vi "createLogFile (SubVI).vi"(8 "TrialInfo":T2={"BlockInfo"={"block #"=0, "block cond"=enum."RHP", "Trial # in block"=0}, "Trial #"=0}, 10 "Subject ID":T1, 11 "directory Path":path) -> (3 "file path out":path)   [LabVIEW 2021]
uses:
  ctrTrialInfo.ctl
  ctrBlockInfo.ctl
  ctrBlockCondition.ctl
  ctlProtocolSubID.ctl
  ctrUnpredictpair.ctl
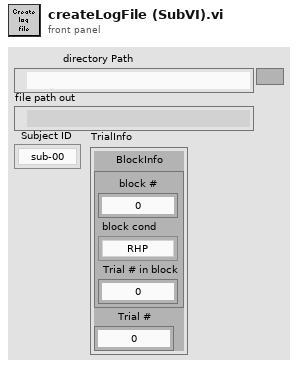
[diagram p1: front panel]
types:
  T1 = typedef "ctlProtocolSubID.ctl" = enum16{"sub-00", "sub-01", "sub-02", "sub-03", "sub-04", "sub-05", "sub-06", "sub-07", "sub-08", "sub-09", "sub-10", "sub-11", "sub-12", "sub-13", "sub-14", "sub-15", "sub-16", "sub-17", "sub-18", "sub-19", "sub-20", "sub-21", "sub-22", "sub-23", "sub-24", "sub-25", "sub-26", "sub-27", "sub-28", "sub-29", "sub-30", "sub-31", "sub-32", "sub-33", "sub-34", "sub-35", "sub-36", "sub-37", "sub-38", "sub-39", "sub-40"}
  T2 = typedef "ctrTrialInfo.ctl" = cluster{"BlockInfo":T3, "Trial #":i32}
  T3 = typedef "ctrBlockInfo.ctl" = cluster{"block #":i32, "block cond":T4, "Trial # in block":i32}
  T4 = typedef "ctrBlockCondition.ctl" = enum16{"famDrop", "preDrop", "famTask", "RHP", "RLD", "RHD", "LHP", "LLD", "LHD", "UR", "UL", "pstDrop"}
  T5 = typedef "ctrUnpredictpair.ctl" = enum16{"HPHP", "LDHP", "HDHP", "HPLD", "HPHD", "LDLD", "HDHD", "HP"}
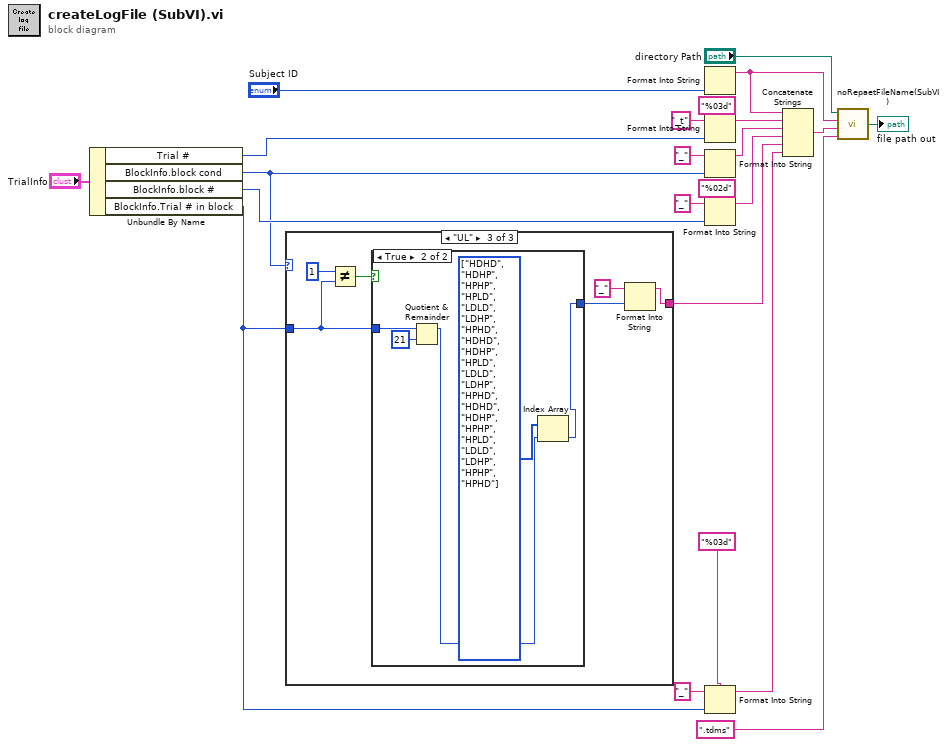
[diagram p0: block diagram]
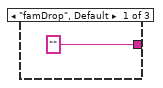
[diagram p2: hidden frame]
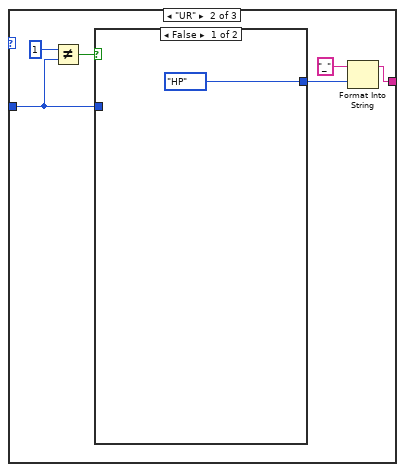
[diagram p3: hidden frame]
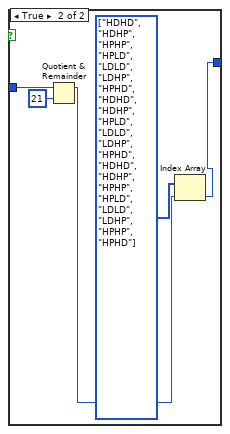
[diagram p4: hidden frame]
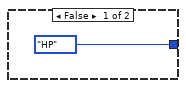
[diagram p5: hidden frame]
diagram:
  n1 = Unbundle By Name("TrialInfo") -> ("Trial #"=w4:i32, "BlockInfo.block cond"=w3:T4, "BlockInfo.block #"=w6:i32, "BlockInfo.Trial # in block"=w1:i32)
  n2 = case shown="\"UL\"" w3 {
    tunnel: ["" ("string") w25 w37] -> w2
    tunnel: w1 -> [_ w30 w42]
    frame "famDrop", Default {
    }
    frame "UR" {
      n3 = Not Equal?(x=1, y=w30) -> (x != y?=w28:bool)
      n4 = case shown="False" w28 {
        tunnel: w30 -> [_ w35]
        tunnel: [ctrUnpredictpair."HP" w32] -> w26
        frame False {
        }
        frame True {
          w34 = T5[] [enum."HDHD", enum."HDHP", enum."HPHP", enum."HPLD", enum."LDLD", enum."LDHP", enum."HPHD", enum."HDHD", enum."HDHP", enum."HPLD", enum."LDLD", enum."LDHP", enum."HPHD", enum."HDHD", enum."HDHP", enum."HPHP", enum."HPLD", enum."LDLD", enum."LDHP", enum."HPHP", enum."HPHD"] items=["HPHP", "LDHP", "HDHP", "HPLD", "HPHD", "LDLD", "HDHD", "HP"] ("Array")
          n5 = Quotient & Remainder(x=w35, y=21) -> (x-y*floor(x/y)=w33:i32)  [unwired: 1 out]
          n6 = Index Array(array=w34, index=w33) -> (element=w32:T5)
        }
      }
      n7 = Format Into String(initial string="_" ("string"), w26) -> (resulting string=w25:string)  [unwired: 2 in, 1 out]
    }
    frame "UL" {
      n8 = Not Equal?(x=1, y=w42) -> (x != y?=w40:bool)
      n9 = case shown="True" w40 {
        tunnel: w42 -> [_ w47]
        tunnel: [ctrUnpredictpair."HP" w44] -> w38
        frame False {
        }
        frame True {
          w46 = T5[] [enum."HDHD", enum."HDHP", enum."HPHP", enum."HPLD", enum."LDLD", enum."LDHP", enum."HPHD", enum."HDHD", enum."HDHP", enum."HPLD", enum."LDLD", enum."LDHP", enum."HPHD", enum."HDHD", enum."HDHP", enum."HPHP", enum."HPLD", enum."LDLD", enum."LDHP", enum."HPHP", enum."HPHD"] items=["HPHP", "LDHP", "HDHP", "HPLD", "HPHD", "LDLD", "HDHD", "HP"] ("Array")
          n10 = Quotient & Remainder(x=w47, y=21) -> (x-y*floor(x/y)=w45:i32)  [unwired: 1 out]
          n11 = Index Array(array=w46, index=w45) -> (element=w44:T5)
        }
      }
      n12 = Format Into String(initial string="_" ("string"), w38) -> (resulting string=w37:string)  [unwired: 2 in, 1 out]
    }
  }
  n13 = Format Into String("Subject ID") -> (resulting string=w19:string)  [unwired: 3 in, 1 out]
  n14 = Format Into String(format string="%03d", initial string="_t", w4) -> (resulting string=w20:string)  [unwired: 1 in, 1 out]
  n15 = Format Into String(initial string="_" ("string"), w3) -> (resulting string=w10:string)  [unwired: 2 in, 1 out]
  n16 = Format Into String(format string="%02d", initial string="_" ("string"), w6) -> (resulting string=w9:string)  [unwired: 1 in, 1 out]
  n17 = Format Into String(format string="%03d", initial string="_" ("string"), w1) -> (resulting string=w8:string)  [unwired: 1 in, 1 out]
  n18 = Concatenate Strings(w19, w20, w10, w9, w2, w8) -> (w17:string)
  n19 = call "noRepaetFileName(SubVI).vi"("ext"=".tdms", "file name"=w17, "subID"=w19, "directory Path"="directory Path") -> ("file path out"=→"file path out":path)  [unwired: 2 in]
